vi "Element2-ManualBuilder.vi"() -> ()   [LabVIEW 2019]
uses:
  <userlib>/LevyLab/Build Support/PostBuildSupport/PostBuildSupport.lvclass
  <vilib>/MakerHub/Toolbox/LMH-Toolbox.lvlib
panel:
  in  "Package Version":string="1.0.0.3"
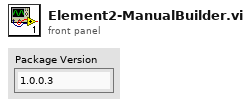
[diagram p1: front panel]
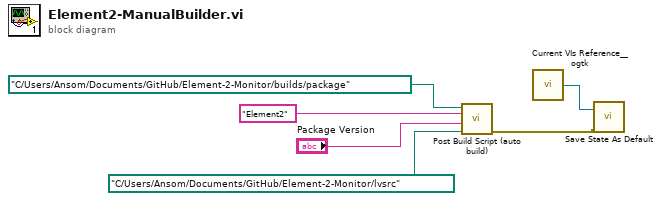
[diagram p0: block diagram]
diagram:
  n1 = call <userlib>:"Post Build Script (auto build).vi"("Package Source Folder"=path "C:/Users/Ansom/Documents/GitHub/Element-2-Monitor/lvsrc", "Package Version"="Package Version", "Product Name"="Element2", "Output Package File Path"=path "C:/Users/Ansom/Documents/GitHub/Element-2-Monitor/builds/package") -> ("error out"=w2:errorcluster)  [unwired: 7 in]
  n2 = call <userlib>:"Current VIs Reference__ogtk.vi"() -> ("Current VI's reference"=w1:refnum<vi>)  [unwired: 5 in]
  n3 = call <vilib>:"Save State As Default.vi"("Error In"=w2, "Target VI"=w1) -> ()  [unwired: 8 in, 2 out]
